vi "test_serpenbot_DDPG_learing.vi"() -> ()   [LabVIEW 2020]
panel:
  out "done":bool
  out "laser control value":dbl[](array[numeric])
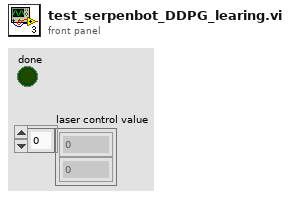
[diagram p1: front panel]
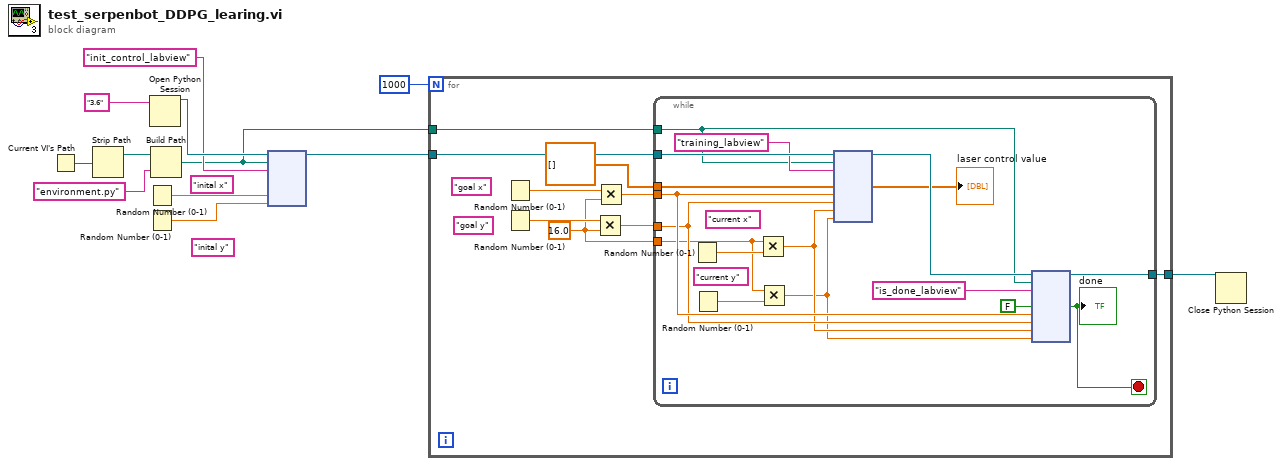
[diagram p0: block diagram]
diagram:
  (unwired) "inital y"
  (unwired) "inital x"
  n1 = Current VI's Path() -> (path=w11:path)
  n2 = Strip Path(path=w11) -> (stripped path=w10:path)  [unwired: 1 out]
  n3 = Random Number (0-1)() -> (number: 0 to 1=w5:dbl)
  n4 = Random Number (0-1)() -> (number: 0 to 1=w4:dbl)
  n5 = Open Python Session(python version="3.6" ("Python version")) -> (session out=w7:refnum<k35>)  [unwired: 2 in, 1 out]
  n6 = Build Path(base path=w10, name or relative path="environment.py") -> (appended path=w1:path)
  n7 = node(w7, w1, "init_control_labview" ("function name"), w5, w4) -> (w3:refnum<k35>)  [unwired: 5 in, 3 out]
  n8 = for {
    N: 1000 -> [_]
    tunnel: w3 -> [w21]
    tunnel: w1 -> [w19]
    tunnel: [w20] -> w2
    w13 = 16.0
    (unwired) "goal y"
    (unwired) "goal x"
    n9 = Random Number (0-1)() -> (number: 0 to 1=w16:dbl)
    n10 = Random Number (0-1)() -> (number: 0 to 1=w14:dbl)
    n11 = Multiply(x=w14, y=w13) -> (x*y=w15:dbl)
    n12 = Multiply(x=w16, y=w13) -> (x*y=w17:dbl)
    n13 = while {
      tunnel: w21 -> [w38]
      tunnel: w17 -> [w34]
      tunnel: w15 -> [w33]
      tunnel: [w30] -> w20
      tunnel: w19 -> [w29]
      tunnel: dbl[] [] -> [w28]
      tunnel: w13 -> [w25]
      stop <- w31 stop-if-true
      (unwired) "current y"
      (unwired) "current x"
      n14 = Random Number (0-1)() -> (number: 0 to 1=w26:dbl)
      n15 = Random Number (0-1)() -> (number: 0 to 1=w24:dbl)
      n16 = Multiply(x=w25, y=w26) -> (x*y=w23:dbl)
      n17 = Multiply(x=w25, y=w24) -> (x*y=w22:dbl)
      n18 = node(w38, w29, "training_labview" ("function name"), w28, w34, w33, w23, w22) -> (w36:refnum<k35>, →"laser control value":dbl[])  [unwired: 5 in, 3 out]
      n19 = node(w36, w29, "is_done_labview" ("function name"), FALSE, w34, w33, w23, w22) -> (w30:refnum<k35>, w31:bool)  [unwired: 5 in, 3 out]
      "done" <- w31
    }
  }
  n20 = Close Python Session(session in=w2) -> ()  [unwired: 1 in, 1 out]
